vi "PWM.vi"() -> ()   [LabVIEW 2016]
uses:
  <vilib>/myRIO/Instrument Drivers/Onboard IO/DIO/typedefs/DIO Reference.ctl
  <vilib>/myRIO/Common/Instrument Driver Framework/Utilities/typedefs/myRIO Generic Hardware Reference.ctl
  <vilib>/myRIO/Common/Instrument Driver Framework/Utilities/typedefs/Hardware Version Enum.ctl
  <vilib>/myRIO/Common/Instrument Driver Framework/Utilities/typedefs/myRIO v1.0 Reference.ctl
  <vilib>/myRIO/Common/Instrument Driver Framework/Utilities/typedefs/Generic FPGA Reference.ctl
  <vilib>/myRIO/Common/Instrument Driver Framework/myRIO v1.0/DIO/typedefs/DIO Channels List.ctl
  <vilib>/myRIO/Common/Instrument Driver Framework/myRIO v1.0/DIO/typedefs/DIO Channels Enum.ctl
  <vilib>/userdefined/High Color/nirio_resource_hc.ctl
  <vilib>/Platform/TimedLoop/XDataNode/timing_clust.ctl
  <vilib>/Platform/TimedLoop/XDataNode/nitl_modes.ctl
  <vilib>/Platform/TimedLoop/XDataNode/wakeup.ctl
  <vilib>/myRIO/Common/Instrument Driver Framework/myRIO v1.0/DIO/vis/myRIO v1.1 Open DIO.vi
  <vilib>/myRIO/Common/Instrument Driver Framework/Utilities/vis/Validate Channels.vi
  <vilib>/myRIO/Common/Instrument Driver Framework/myRIO v1.0/DIO/vis/myRIO v1.0 Reserve DIO.vi
  <vilib>/myRIO/Common/Instrument Driver Framework/myRIO v1.0/DIO/vis/myRIO v1.0 Close DIO.vi
  <vilib>/myRIO/Common/Instrument Driver Framework/myRIO v1.0/Resource Manager/vis/myRIO v1.0 Reserve Channel List.vi
  <vilib>/myRIO/Common/Instrument Driver Framework/myRIO v1.0/DIO/vis/myRIO v1.0 Build MUX Configuration DIO.vi
  <vilib>/myRIO/Common/Instrument Driver Framework/myRIO v1.0/DIO/vis/myRIO v1.0 Unreserve DIO.vi
  <vilib>/myRIO/Common/Instrument Driver Framework/myRIO v1.0/Resource Manager/vis/myRIO v1.0 Reserve Channel.vi
  <vilib>/myRIO/Common/Instrument Driver Framework/myRIO v1.0/Resource Manager/vis/myRIO v1.0 Unreserve Channel.vi
  <vilib>/myRIO/Common/Instrument Driver Framework/myRIO v1.0/Resource Manager/vis/myRIO v1.0 Create Configuration List.vi
  <vilib>/myRIO/Common/Instrument Driver Framework/myRIO v1.0/Resource Manager/vis/myRIO v1.0 Unreserve Channel List.vi
  <vilib>/myRIO/Common/Instrument Driver Framework/myRIO v1.0/Resource Manager/vis/myRIO v1.0 Build Mutex Name.vi
  <vilib>/Utility/VariantDataType/GetNumericInfo.vi
  <vilib>/Utility/error.llb/Error Cluster From Error Code.vi
  <vilib>/myRIO/Common/Instrument Driver Framework/myRIO v1.0/myRIO v1.1 Open.vi
  <vilib>/myRIO/Common/Instrument Driver Framework/Utilities/vis/IO Manager.vi
  <vilib>/myRIO/Common/Instrument Driver Framework/Utilities/vis/Configuration Manager.vi
  <vilib>/myRIO/Common/Instrument Driver Framework/myRIO v1.0/Resource Manager/vis/myRIO v1.0 Configure IO.vi
  <vilib>/myRIO/Common/Instrument Driver Framework/myRIO v1.0/myRIO v1.0 Close.vi
  <vilib>/myRIO/Common/Instrument Driver Framework/myRIO v1.0/DIO/vis/myRIO v1.0 Write DIO.vi
  <vilib>/myRIO/Common/Instrument Driver Framework/myRIO v1.0/DIO/vis/myRIO v1.0 Read DIO.vi
  <vilib>/myRIO/Common/Instrument Driver Framework/myRIO v1.0/DIO/vis/myRIO v1.0 Shutdown DIO.vi
  <vilib>/myRIO/Instrument Drivers/Onboard IO/DIO/vis/myRIO DIO Open.xnode
  <vilib>/Platform/TimedLoop/XDataNode/XDataNode.xnode
  <vilib>/myRIO/Instrument Drivers/Onboard IO/DIO/DIO.lvlib
  <vilib>/Platform/TimedLoop/XDataNode/XDNodeRunTimeDep.lvlib
panel:
  out "Numeric":i32
  out "Array":u32[](array[numeric])
  out "Array 2":u32[](array[numeric])
  out "Finished Late? [i-1]":bool
  out "Error":errorcluster
  out "source out":string
  out "error out":errorcluster
  in  "error in (no error)":errorcluster
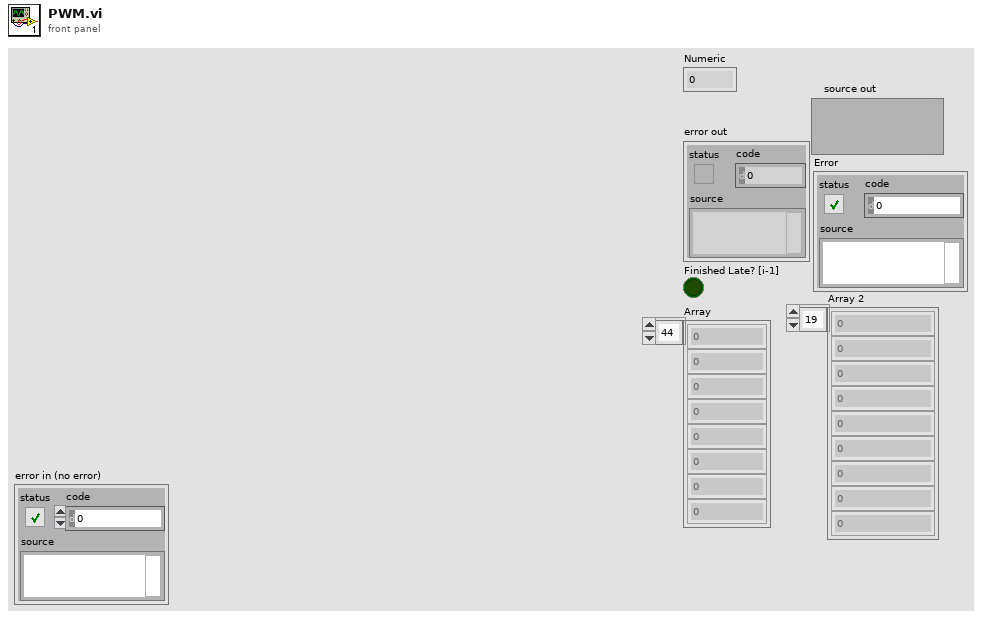
[diagram p1: front panel]
types:
  T1 = typedef "nirio_resource_hc.ctl" = tag
  T2 = typedef "Hardware Version Enum.ctl" = enum16{"Unknown", "myRIO-1900", "myRIO-1950", "roboRIO", "NI ELVIS RIO CM"}
  T3 = typedef "XDNodeRunTimeDep.lvlib/timing_clust.ctl" = cluster{"Expected End [f-1]":u64, "Actual End [f-1]":u64, "Finished Late? [f-1]":bool, "Expected End [i-1]":u64, "Actual End [i-1]":u64, "Finished Late? [i-1]":bool, "Expected Start [i]":u64, "Actual Start [i]":u64, "Expected Start [f]":u64, "Actual Start [f]":u64, "Source Name":string, "Structure Name":string, "Period":i64, "Deadline":i64, "Offset":i64, "Start":i64, "Priority":i32, "Timeout":i32, "Mode":T4, "Wakeup Reason":T5, "Error":errorcluster, "Source Type":string, "Secondary Source Type":string, "Global End Time":u64, "Global Start Time":u64, "Frame Duration":u64, "Iteration Duration":u64, "Assigned CPU":i32, "I/O Scan Engine Mode":u32}
  T4 = typedef "XDNodeRunTimeDep.lvlib/nitl_modes.ctl" = enum32{"No Change", "Process missed periods, maintain original phase", "Discard missed periods, maintain original phase", "Process missed periods, ignore original phase", "Discard missed periods, ignore original phase"}
  T5 = typedef "XDNodeRunTimeDep.lvlib/wakeup.ctl" = enum32{"Normal", "Aborted", "Asynchronous wakeup", "Timing source error", "Timed loop error", "Timeout"}
  T6 = typedef "DIO.lvlib/DIO Reference.ctl" = cluster{"myRIO Reference":T7, "DIO Channels List":T10}
  T7 = typedef "myRIO Generic Hardware Reference.ctl" = cluster{"myRIO Model":T2, "myRIO Hardware Reference":T8}
  T8 = typedef "myRIO v1.0 Reference.ctl" = cluster{"Generic FPGA Reference":T9, "Allow multiple opens":bool}
  T9 = typedef "Generic FPGA Reference.ctl" = refnum<k20>
  T10 = typedef "DIO Channels List.ctl" = T11[]
  T11 = typedef "DIO Channels Enum.ctl" = enum16{"Not Connected", "C/DIO0", "C/DIO1", "C/DIO2", "C/DIO3", "C/DIO4", "C/DIO5", "C/DIO6", "C/DIO7", "A/DIO0", "A/DIO1", "A/DIO2", "A/DIO3", "A/DIO4", "A/DIO5", "A/DIO6", "A/DIO7", "A/DIO8", "A/DIO9", "A/DIO10", "A/DIO11", "A/DIO12", "A/DIO13", "A/DIO14", "A/DIO15", "B/DIO0", "B/DIO1", "B/DIO2", "B/DIO3", "B/DIO4", "B/DIO5", "B/DIO6", "B/DIO7", "B/DIO8", "B/DIO9", "B/DIO10", "B/DIO11", "B/DIO12", "B/DIO13", "B/DIO14", "B/DIO15", "LED0", "LED1", "LED2", "LED3", "Button0", "DIO/DIO0", "DIO/DIO1", "DIO/DIO2", "DIO/DIO3", "DIO/DIO4", "DIO/DIO5", "DIO/DIO6", "DIO/DIO7", "DIO/DIO8", "DIO/DIO9", "SPI/CS0", "SPI/CS1", "SPI/CS2", "SPI/CS3", "LED RADIO (Green)", "LED RADIO (Red)", "LED COMM (Green)", "LED COMM (Red)", "LED MODE (Green)", "LED MODE (Red)"}
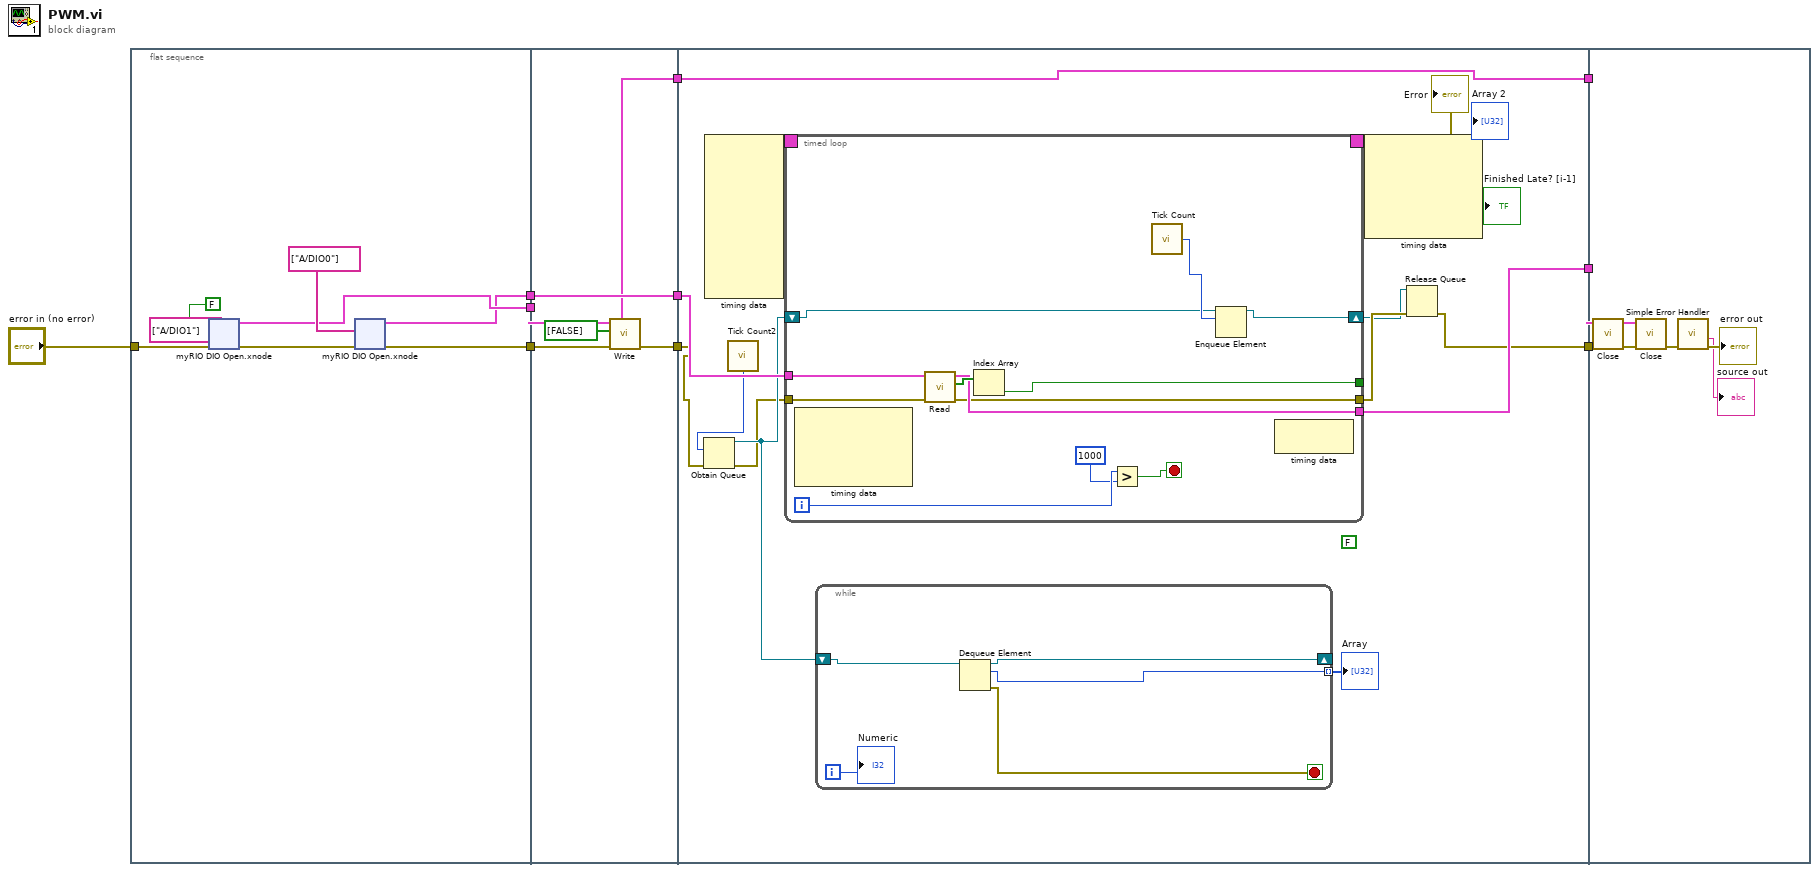
[diagram p0: block diagram]
diagram:
  n1 = flat-sequence {
    tunnel: "error in (no error)" -> [w18]
    tunnel: [w13] -> w9
    tunnel: [w12] -> w8
    tunnel: [w11] -> w6
    tunnel: w9 -> [w56]
    tunnel: w8 -> [w55]
    tunnel: [w53] -> w7
    tunnel: w6 -> [w53]
    tunnel: [w52] -> w5
    tunnel: [w51] -> w3
    tunnel: w7 -> [w68]
    tunnel: w5 -> [w61]
    tunnel: [w71] -> w4
    tunnel: w3 -> [w71]
    tunnel: [w67] -> w2
    tunnel: [w58] -> w1
    tunnel: w4 -> [w101]
    tunnel: w2 -> [w97]
    tunnel: w1 -> [w96]
    frame #0 {
      n2 = xnode "myRIO DIO Open.xnode"("error in (no error)"=w18, "Allow multiple opens?"=FALSE, "Channel Names"=tag[] ["A/DIO1"]) -> ("error out"=w15:errorcluster, "DIO Ref Out"=w13:T6)
      n3 = xnode "myRIO DIO Open.xnode"("error in (no error)"=w15, "Channel Names"=tag[] ["A/DIO0"]) -> ("error out"=w12:errorcluster, "DIO Ref Out"=w11:T6)  [unwired: 1 in]
    }
    frame #1 {
      n4 = call <vilib>:"Write.vi"("error in (no error)"=w55, "Values"=bool[] [FALSE], "DIO Ref In"=w56) -> ("error out"=w52:errorcluster, "DIO Ref Out"=w51:T6)  [unwired: 6 in]
    }
    frame #2 {
      (unwired) FALSE
      n5 = node-c288() -> (w70:T3)  [unwired: 9 in]
      n6 = call "Tick Count2"() -> ("Tick Count(uSec)"=w63:u32)
      n7 = Obtain Queue(element data type=w63, error in (no error)=w61) -> (queue out=w64:refnum<queue>, error out=w60:errorcluster)  [unwired: 3 in, 1 out]
      n8 = timed-loop {
        timing: w70 -> [_]
        timing-out: [_] -> w69
        tunnel: w60 -> [w88]
        tunnel: w68 -> [w87]
        tunnel: [w85] -> w67
        tunnel: [w84] -> w59
        tunnel: [w80] -> _
        shift-right: [w78] -> w57
        shift-left: w64 -> [w77]
        i -> [w83]
        stop <- w81 stop-if-true
        n9 = node-c288() -> ()  [unwired: 1 in, 4 out]
        n10 = call <vilib>:"Read.vi"("error in (no error)"=w88, "DIO Ref In"=w87) -> ("error out"=w84:errorcluster, "Values"=w86:bool[], "DIO Ref Out"=w85:T6)  [unwired: 7 in]
        n11 = Index Array(array=w86) -> (element=w80:bool)  [unwired: 1 in]
        n12 = Greater?(x=w83, y=1000) -> (0:w81:bool)
        n13 = call "Tick Count"() -> ("Tick Count(uSec)"=w79:u32)
        n14 = Enqueue Element(queue=w77, element=w79) -> (queue out=w78:refnum<queue>)  [unwired: 2 in, 2 out]
        n15 = node-c288() -> ()  [unwired: 1 in, 1 out]
      }
      n16 = while {
        shift-right: [w74] -> _
        shift-left: w64 -> [w76]
        tunnel: [w73] -> w62 mode=indexing
        i -> [w72]
        stop <- w75 stop-if-true
        n17 = Dequeue Element(queue=w76) -> (queue out=w74:refnum<queue>, element=w73:u32, error out=w75:errorcluster)  [unwired: 2 in, 1 out]
        "Numeric" <- w72
      }
      "Array" <- w62
      n18 = node-c288(w69) -> (→"Error":errorcluster, →"Finished Late? [i-1]":bool)  [unwired: 3 out]
      n19 = Release Queue(queue=w57, error in (no error)=w59) -> (error out=w58:errorcluster)  [unwired: 1 in, 2 out]
    }
    frame #3 {
      n20 = call <vilib>:"Close.vi"("error in (no error)"=w96, "DIO Ref In"=w97) -> ("error out"=w100:errorcluster)  [unwired: 9 in]
      n21 = call <vilib>:"Close.vi"("error in (no error)"=w100, "DIO Ref In"=w101) -> ("error out"=w99:errorcluster)  [unwired: 9 in]
      n22 = call <vilib>:"Simple Error Handler.vi"("error in (no error)"=w99) -> ("source out"=→"source out":string, "error out"=→"error out":errorcluster)  [unwired: 4 in, 3 out]
    }
  }
